vi "Loadcell Match.vi"(6 "Initialize":bool, 9 "Set Tension":dbl[](array[numeric]), 10 "Mes Tension":dbl[](array[numeric]), 11 "Next Tension Error":dbl[](array[numeric])) -> (2 "Tension Error":dbl[](array[numeric]), 3 "Filtered Tension":dbl[](array[numeric]))   [LabVIEW 2021]
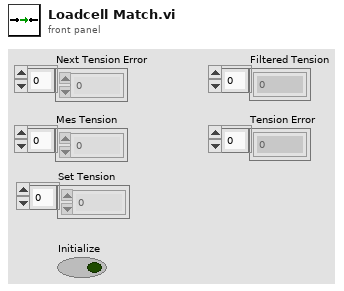
[diagram p1: front panel]
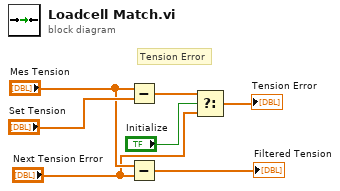
[diagram p0: block diagram]
diagram:
  # "Tension Error"
  n1 = Subtract(x="Mes Tension", y="Set Tension") -> (x-y=w6:dbl[])
  n2 = Subtract(x="Mes Tension", y="Next Tension Error") -> (x-y=→"Filtered Tension":dbl[])
  n3 = Select(t=w6, s="Initialize", f="Next Tension Error") -> (s? t:f=→"Tension Error":dbl[])
